vi "MFC MAXtest FPGA.vi"() -> ()   [LabVIEW 2011]
uses:
  <vilib>/rvi/eio/common/nirviEmuTemplateMethod_errors.vi
  <vilib>/eio/EIOMethodNode/EIOMethodNode.xnode
panel:
  out "Timed Out":bool
  in  "array":u8[](array[numeric])=[65, 48, 48, 48, 48, 48, 13]
  # "32000"
  # "64000"
  # "66.....73"
  # "65\n48\n48\n48\n48\n48\n13"
  # "64\n51  \n50\n48\n48\n48\n13"
  # "65\n54\n52\n52\n48\n48\n13"
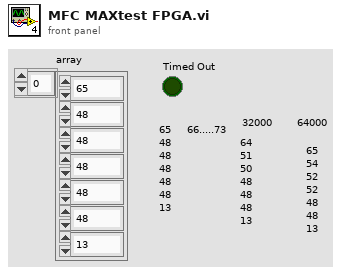
[diagram p1: front panel]
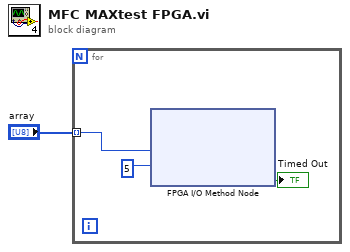
[diagram p0: block diagram]
diagram:
  n1 = for {
    tunnel: "array" -> [w3] mode=indexing
    n2 = xnode "FPGA I/O Method Node"("Data"=w3, "Timeout (ms)"=5) -> ("Timed Out"=→"Timed Out":bool)  [unwired: 2 in, 2 out]
  }
